vi "ALARM Clear.vi"(8 "error in (no error)":errorcluster, 10 "Message Data":variant, 11 "Data Cluster":T1={"LOG REF"=refnum, "Writer Queue"=refnum, "Log Path"=path "", "UPS standby"=FALSE, "status code"=5001, "SP"=[], "Over Sens Status"=[]}) -> (0 "error out":errorcluster, 3 "Data Cluster out":T1={"LOG REF"=refnum, "Writer Queue"=refnum, "Log Path"=path "", "UPS standby"=FALSE, "status code"=5001, "SP"=[], "Over Sens Status"=[]})   [LabVIEW 2020, in "QCT ALARM.lvlib"]
uses:
  QCT ALARM.lvlib
  ALARM Configuration.ctl
  support/Message Queue/Message Cluster.ctl
  support/Message Queue/Message Queue.lvlib
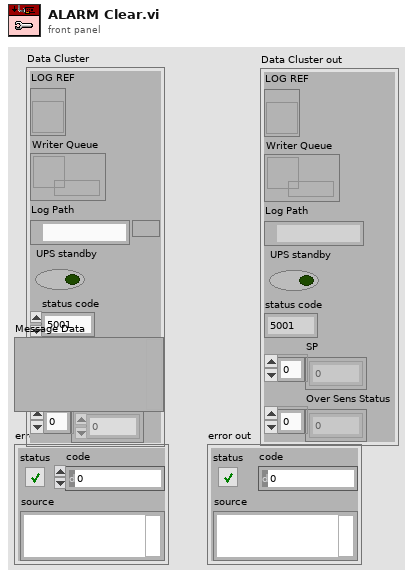
[diagram p1: front panel]
types:
  T1 = typedef "QCT ALARM.lvlib/ALARM Configuration.ctl" = cluster{"LOG REF":refnum<vi>, "Writer Queue":refnum<queue>, "Log Path":path, "UPS standby":bool, "status code":i32, "SP":dbl[], "Over Sens Status":dbl[]}
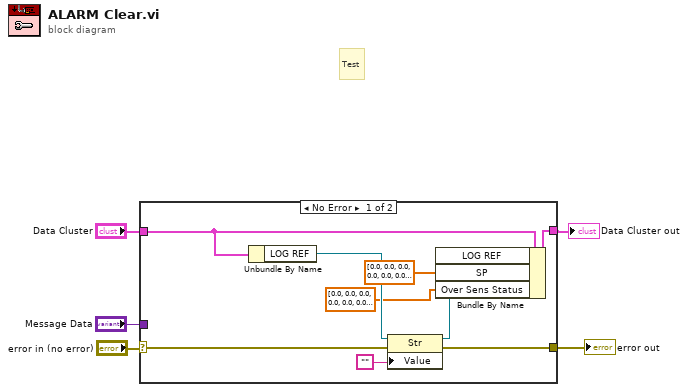
[diagram p0: block diagram]
diagram:
  # "Test"
  n1 = case shown="No Error" "error in (no error)" {
    selector: "error in (no error)" -> [w9 w15]
    tunnel: [w14 w16] -> w4
    tunnel: "Data Cluster" -> [w13 w16]
    tunnel: [w12 w15] -> w3
    tunnel: "Message Data" -> [_ _]
    frame No Error {
      n2 = Unbundle By Name(w13) -> ("LOG REF"=w11:refnum<vi>)
      n3 = property class="Str"(reference=w11, error in=w9, "Value"="") -> (reference out=w10:refnum<vi>, error out=w12:errorcluster)
      n4 = Bundle By Name(cluster=w13, "LOG REF"=w10, "SP"=dbl[] [0.0, 0.0, 0.0, 0.0, 0.0, 0.0, 0.0, 0.0, 0.0, 0.0], "Over Sens Status"=dbl[] [0.0, 0.0, 0.0, 0.0, 0.0, 0.0, 0.0, 0.0, 0.0, 0.0, 0.0, 0.0, 0.0, 0.0, 0.0, 0.0, 0.0, 0.0, 0.0, 0.0, 0.0, 0.0, 0.0, 0.0, 0.0, 0.0, 0.0, 0.0, 0.0, 0.0, 0.0, 0.0, 0.0, 0.0, 0.0, 0.0, 0.0, 0.0, 0.0, 0.0, 0.0, 0.0, 0.0, 0.0, 0.0, 0.0, 0.0, 0.0, 0.0, 0.0, 0.0, 0.0, 0.0, 0.0, 0.0, 0.0, 0.0, 0.0, 0.0, 0.0, 0.0, 0.0, 0.0, 0.0, 0.0, 0.0, 0.0, 0.0, 0.0, 0.0, 0.0, 0.0, 0.0, 0.0, 0.0, 0.0, 0.0, 0.0, 0.0, 0.0] ("SP")) -> (w14:T1)
    }
    frame Error {
    }
  }
  "error out" <- w3
  "Data Cluster out" <- w4
